vi "set_query infusion rate.vi"(0 "VISA resource name":refnum<visa-resource-name>, 5 "Query?":bool, 7 "Rate":dbl=1.0 min=0.0 max=999.0 step=0.001, 9 "Flow Rate Units":u32(ring)=1 items=["milliliters per hour (ml/hr)", "milliliters per minute (ml/min)", "microliters per hour (ul/hr)", "microliters per minute (ul/min)", "microliters per second (ul/sec)", "nanoliters per second (nl/sec)"], 11 "error in (no error)":errorcluster) -> (4 "VISA resource name out":refnum<visa-resource-name>, 6 "Output infusion rate":string, 15 "error out":errorcluster)   [LabVIEW 2016]
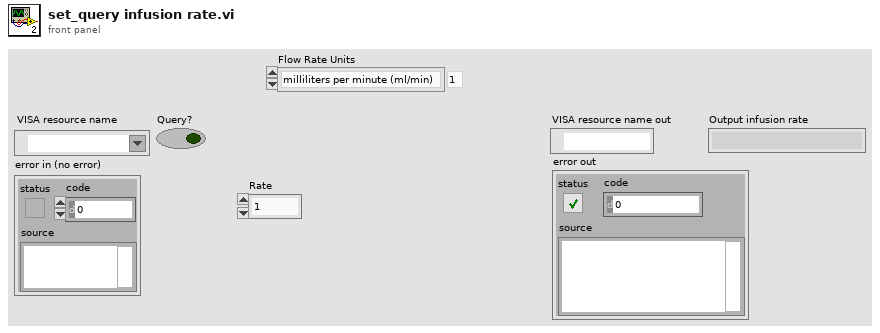
[diagram p1: front panel]
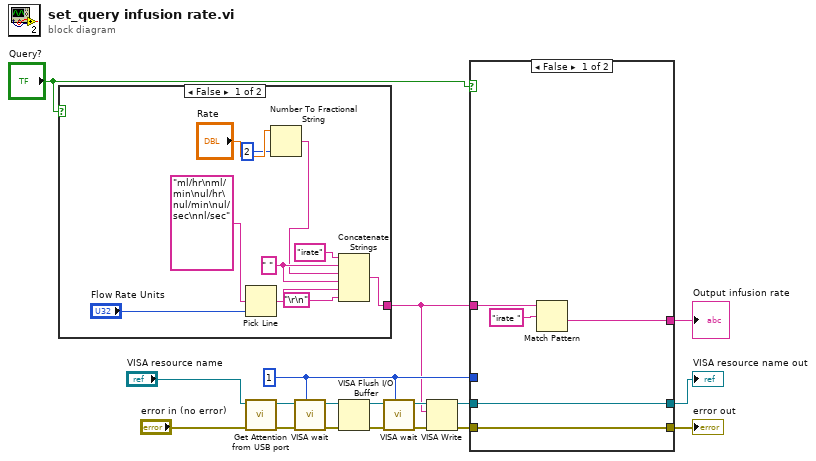
[diagram p0: block diagram]
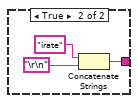
[diagram p2: hidden frame]
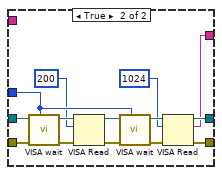
[diagram p3: hidden frame]
diagram:
  w4 = u32 1 ("milliseconds to wait")
  n1 = case shown="False" "Query?" {
    tunnel: [w24 w29] -> w1
    frame False {
      w27 = " " ("string")
      n2 = Pick Line(multi-line string="ml/hr\nml/min\nul/hr\nul/min\nul/sec\nnl/sec", line index="Flow Rate Units") -> (output string=w26:string)  [unwired: 1 in]
      n3 = Number To Fractional String(number="Rate", precision (6)=i16 2) -> (F-format string=w20:string)  [unwired: 2 in]
      n4 = Concatenate Strings("irate" ("string"), w27, w20, w27, w26, "\r\n") -> (w24:string)
    }
    frame True {
      n5 = Concatenate Strings("irate" ("string"), "\r\n") -> (w29:string)
    }
  }
  n6 = call "Get Attention from USB port.vi"("error in (no error)"="error in (no error)", "VISA resource name"="VISA resource name") -> ("error out"=w15:errorcluster, "VISA resource name out"=w16:refnum<visa-resource-name>)  [unwired: 8 in]
  n7 = call <userlib>:"VISA wait.vi"("VISA resource name"=w16, "error in (no error)"=w15, "milliseconds to wait"=w4) -> ("VISA resource name out"=w13:refnum<visa-resource-name>, "error out"=w14:errorcluster)  [unwired: 6 in]
  n8 = VISA Flush I/O Buffer(VISA resource name=w13, error in (no error)=w14) -> (VISA resource name out=w12:refnum<visa-resource-name>, error out=w11:errorcluster)  [unwired: 1 in]
  n9 = call <userlib>:"VISA wait.vi"("VISA resource name"=w12, "error in (no error)"=w11, "milliseconds to wait"=w4) -> ("VISA resource name out"=w9:refnum<visa-resource-name>, "error out"=w10:errorcluster)  [unwired: 6 in]
  n10 = VISA Write(VISA resource name=w9, write buffer=w1, error in (no error)=w10) -> (VISA resource name out=w8:refnum<visa-resource-name>, error out=w7:errorcluster)  [unwired: 1 out]
  n11 = case shown="False" "Query?" {
    tunnel: w8 -> [w36 w50]
    tunnel: w7 -> [w35 w49]
    tunnel: [w36 w42] -> w6
    tunnel: [w35 w41] -> w5
    tunnel: w4 -> [_ w40]
    tunnel: [w33 w37] -> w3
    tunnel: w1 -> [w34 _]
    frame False {
      n12 = Match Pattern(string=w34, regular expression="irate ") -> (after substring=w33:string)  [unwired: 1 in, 3 out]
    }
    frame True {
      n13 = call <userlib>:"VISA wait.vi"("VISA resource name"=w50, "error in (no error)"=w49, "milliseconds to wait"=w40) -> ("VISA resource name out"=w47:refnum<visa-resource-name>, "error out"=w48:errorcluster)  [unwired: 6 in]
      n14 = VISA Read(VISA resource name=w47, byte count=u32 200, error in (no error)=w48) -> (VISA resource name out=w46:refnum<visa-resource-name>, error out=w45:errorcluster)  [unwired: 2 out]
      n15 = call <userlib>:"VISA wait.vi"("VISA resource name"=w46, "error in (no error)"=w45, "milliseconds to wait"=w40) -> ("VISA resource name out"=w43:refnum<visa-resource-name>, "error out"=w44:errorcluster)  [unwired: 6 in]
      n16 = VISA Read(VISA resource name=w43, byte count=u32 1024, error in (no error)=w44) -> (VISA resource name out=w42:refnum<visa-resource-name>, read buffer=w37:string, error out=w41:errorcluster)  [unwired: 1 out]
    }
  }
  "VISA resource name out" <- w6
  "error out" <- w5
  "Output infusion rate" <- w3
